vi "Add File Path to VI Title.vi"(6 "Add Asterisk?":bool, 8 "Error In":errorcluster, 9 "VI Title":string, 10 "File Path":path, 11 "VI Refnum":refnum<vi>) -> (0 "Error Out":errorcluster)   [LabVIEW 2021, in "GUI.lvlib"]
uses:
  GUI.lvlib
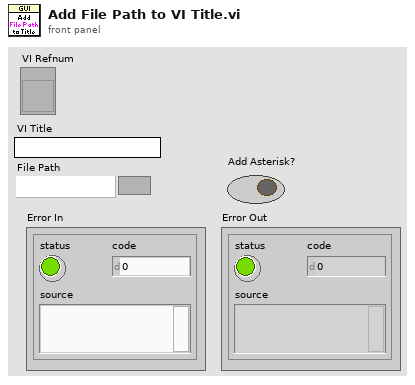
[diagram p1: front panel]
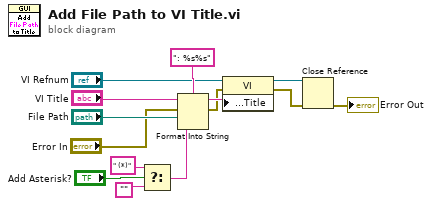
[diagram p0: block diagram]
diagram:
  n1 = Select(t=" (*)" ("format string"), s="Add Asterisk?", f="") -> (s? t:f=w2:string)
  n2 = Format Into String(format string=": %s%s", initial string="VI Title", error in="Error In", "File Path", w2) -> (resulting string=w13:string, error out=w6:errorcluster)
  n3 = property class="VI"(reference="VI Refnum", error in=w6, "Front Panel.Title"=w13) -> (reference out=w9:refnum<vi>, error out=w8:errorcluster)
  n4 = Close Reference(reference=w9, error in (no error)=w8) -> (error out=→"Error Out":errorcluster)
